vi "Read I8 1D Value.vi"(8 "error in (no error)":errorcluster, 11 "Numeric in":refnum<class "Abs_Numeric_1D.lvclass">) -> (0 "error out":errorcluster, 2 "I8":i8[](array[numeric]), 3 "Numeric out":refnum<class "Abs_Numeric_1D.lvclass">)   [LabVIEW 2021, in "Abs_Numeric_1D.lvclass"]
uses:
  Abs_Numeric_1D.lvclass
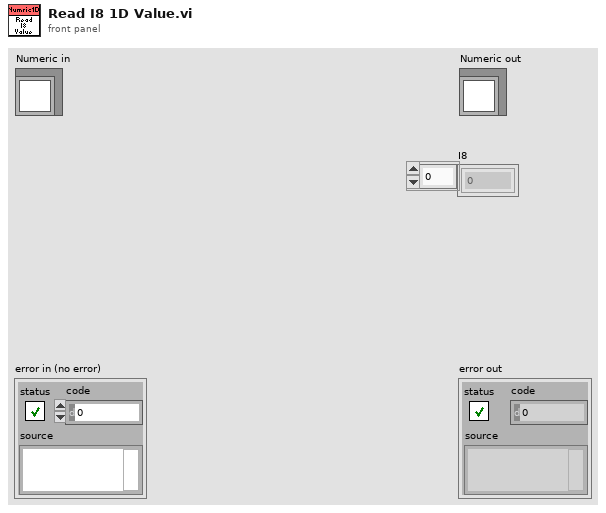
[diagram p1: front panel]
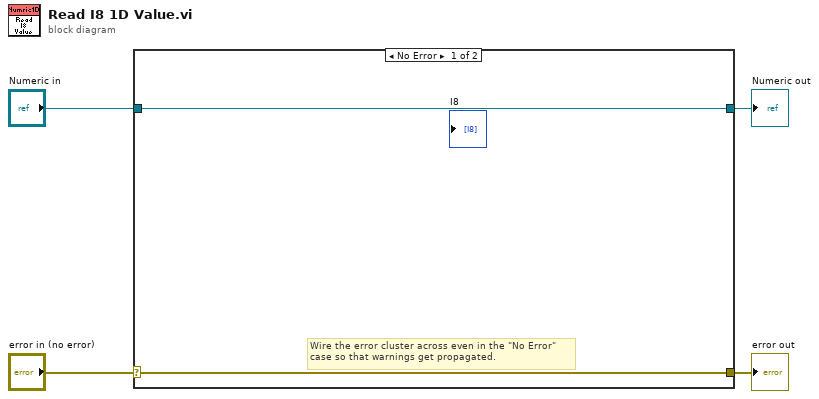
[diagram p0: block diagram]
diagram:
  n1 = case shown="No Error" "error in (no error)" {
    selector: "error in (no error)" -> [w5 w8]
    tunnel: [w5 w8] -> w3
    tunnel: [w6 w7] -> w1
    tunnel: "Numeric in" -> [w6 w7]
    frame No Error {
      # "Wire the error cluster across even in the \"No Error\"\ncase so that warnings get propagated."
    }
    frame Error {
    }
  }
  "error out" <- w3
  "Numeric out" <- w1
